vi "Read datatype.vi"(8 "error in (no error)":errorcluster, 11 "DoublePointer in":refnum<class "DoublePointer.lvclass">) -> (0 "error out":errorcluster, 2 "datatype":string, 3 "DoublePointer out":refnum<class "DoublePointer.lvclass">)   [LabVIEW 2014, in "DoublePointer.lvclass"]
uses:
  DoublePointer.lvclass
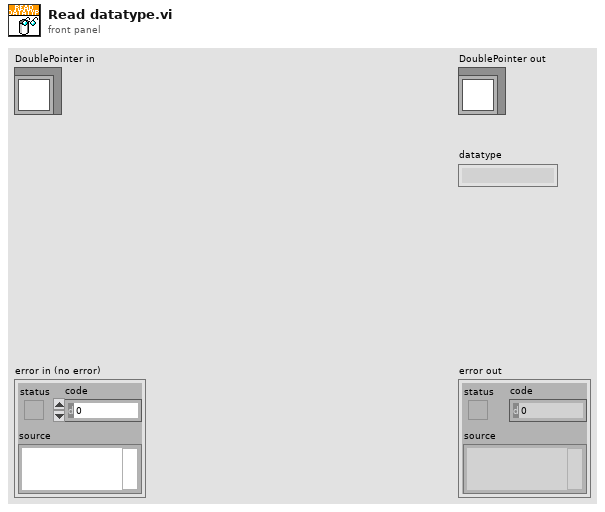
[diagram p1: front panel]
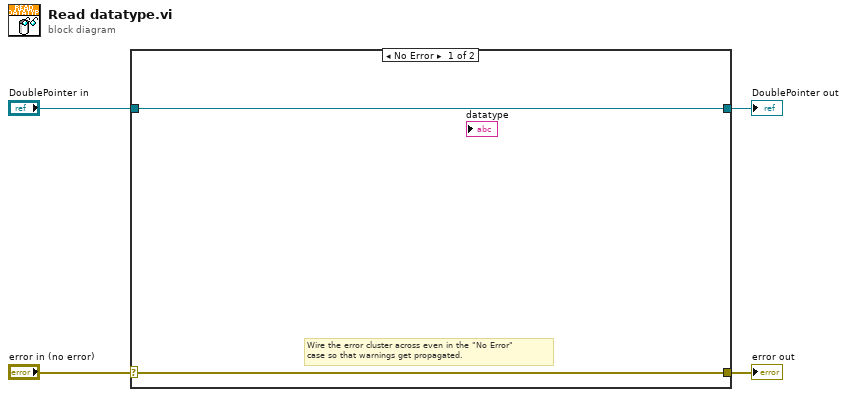
[diagram p0: block diagram]
diagram:
  n1 = case shown="No Error" "error in (no error)" {
    selector: "error in (no error)" -> [w5 w8]
    tunnel: [w5 w8] -> w3
    tunnel: [w6 w7] -> w1
    tunnel: "DoublePointer in" -> [w6 w7]
    frame No Error {
      # "Wire the error cluster across even in the \"No Error\"\ncase so that warnings get propagated."
    }
    frame Error {
    }
  }
  "error out" <- w3
  "DoublePointer out" <- w1
